vi "Send Nested View Insert Front Panel.vi"(8 "error in (no error)":errorcluster, 10 "View Index":i32, 11 "ExampleViewManager in":refnum<class "ExampleViewManager.lvclass">) -> (0 "error out":errorcluster, 3 "ExampleViewManager out":refnum<class "ExampleViewManager.lvclass">)   [LabVIEW 2017, in "MVA Example.lvlib" / "ExampleViewManager.lvclass"]
uses:
  ExampleViewManager.lvclass
  C:/Program Files (x86)/National Instruments/LabVIEW 2017/vi.lib/Composed Systems/MVA Framework/Framework/IViewManager/IViewManager/IViewManager.lvclass
  <vilib>/Composed Systems/MVA Framework/Framework/IViewManager/IViewManager/IViewManager.lvclass/IViewManager.ctl
  ExampleViewManager.lvclass/ExampleViewManager.ctl
  <vilib>/Composed Systems/MVA Framework/Framework/IViewable/IViewable Messages/Insert Front Panel Msg/Insert Front Panel Msg.lvclass/Insert Front Panel Msg.ctl
  <vilib>/ActorFramework/Message Enqueuer/Message Enqueuer.lvclass/Message Enqueuer.ctl
  <vilib>/ActorFramework/Message Enqueuer/Enqueue.vi
  <vilib>/Composed Systems/MVA Framework/Framework/IViewable/IViewable Messages/Insert Front Panel Msg/Insert Front Panel Msg.lvclass
  C:/Program Files (x86)/National Instruments/LabVIEW 2017/vi.lib/ActorFramework/Message/Message.lvclass
  <vilib>/ActorFramework/Message Priority Queue/Priority Enqueue.vi
  <vilib>/Composed Systems/MVA Framework/Framework/IViewManager/IViewManager/IViewManager.lvclass
  <vilib>/Composed Systems/MVA Framework/Framework/IViewable/ProtectedSubpanel/ProtectedSubpanel.lvclass
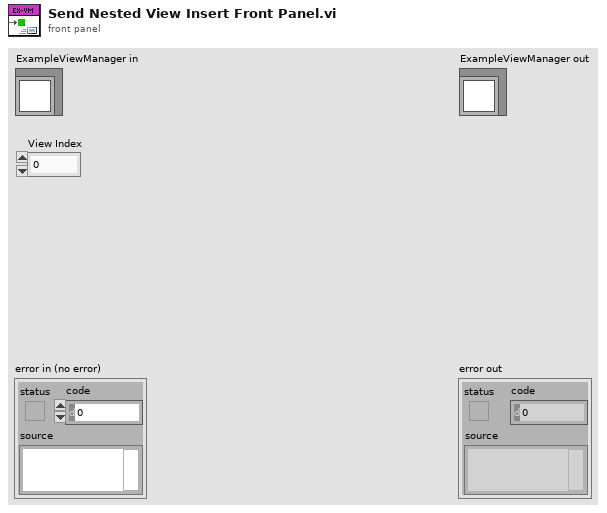
[diagram p1: front panel]
types:
  T1 = typedef "IViewable.lvlib/ProtectedSubpanel.lvclass/Protected Subpanel Reference.ctl" = refnum<data-value>
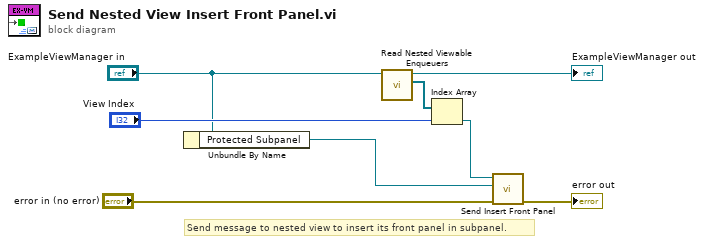
[diagram p0: block diagram]
diagram:
  # "Send message to nested view to insert its front panel in subpanel."
  n1 = Unbundle By Name("ExampleViewManager in") -> ("Protected Subpanel"=w3:T1)
  n2 = call <vilib>:"Read Nested Viewable Enqueuers.vi"("IViewManager in"="ExampleViewManager in") -> ("Nested Viewable Enqueuers"=w7:refnum<class "Message Enqueuer.lvclass">[])  [unwired: 9 in, 1 out]
  n3 = Index Array(array=w7, index="View Index") -> (element=w6:refnum<class "Message Enqueuer.lvclass">)
  n4 = call <vilib>:"Send Insert Front Panel.vi"("error in (no error)"="error in (no error)", "Protected Subpanel"=w3, "Message Enqueuer"=w6) -> ("error out"=→"error out":errorcluster)  [unwired: 7 in, 1 out]
  "ExampleViewManager out" <- "ExampleViewManager in"
